vi "Add Starting Buffer Index.vi"(8 "error in":errorcluster, 10 "starting buffer index":i32, 11 "custom device":T1=18446744073709551615 format="%.0x") -> (0 "error out":errorcluster, 3 "custom device out":T1 format="%.0x")   [LabVIEW 2020, in "AIM MIL-STD-1553 Scripting.lvlib"]
doc: "Adds or replaces the <b>starting buffer index</b>."
uses:
  AIM MIL-STD-1553 Scripting.lvlib
  <vilib>/NI VeriStand/Custom Device API/Custom Device Item Ref.ctl
  Constants.vi
  <vilib>/NI VeriStand/Custom Device API/Custom Device API.lvlib
  <vilib>/NI VeriStand/Custom Device API/Set Item Property (U16).vi
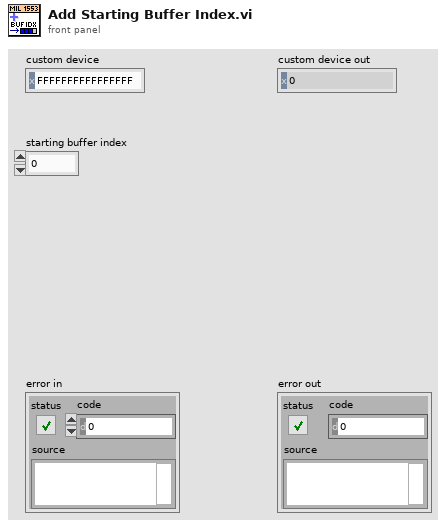
[diagram p1: front panel]
types:
  T1 = typedef "Custom Device API.lvlib/Custom Device Item Ref.ctl" = u64
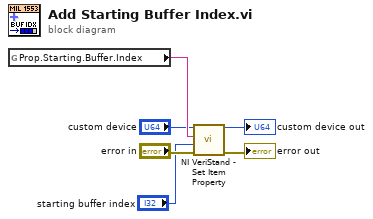
[diagram p0: block diagram]
diagram:
  n1 = global read "Constants.vi" "Prop.Starting.Buffer.Index"() -> (w6:string)
  n2 = call-poly <vilib>:"NI VeriStand - Set Item Property.vi"("error in (no error)"="error in", "Value"="starting buffer index", "Property Name"=w6, "Item Ref in"="custom device") -> ("error out"=→"error out":errorcluster, "Item Ref out"=→"custom device out":T1)  [unwired: 5 in, 1 out]
